vi "add rows_2 (SubVI).vi"(1 "array in":dbl[][](array[numeric])) -> (0 "array out":dbl[](array[numeric]))   [LabVIEW 2009]
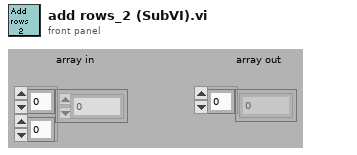
[diagram p1: front panel]
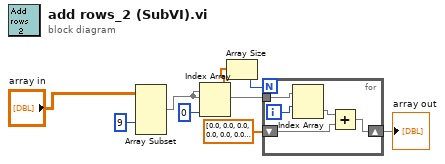
[diagram p0: block diagram]
diagram:
  n1 = Array Subset(array="array in", index (col)=9 ("index")) -> (w3:dbl[][])  [unwired: 3 in]
  n2 = Index Array(array=w3, index (col)=0 ("disabled index (col)")) -> (element=w5:dbl[])  [unwired: 1 in]
  n3 = Array Size(array=w5) -> (size(s)=w6:i32)
  n4 = for {
    N: w6 -> [_]
    tunnel: w3 -> [w13]
    shift-right: [w10] -> w1
    shift-left: dbl[] [0.0, 0.0, 0.0, 0.0, 0.0, 0.0, 0.0, 0.0, 0.0] -> [w9]
    i -> [w12]
    n5 = Index Array(array=w13, index (row)=w12) -> (element=w11:dbl[])  [unwired: 1 in]
    n6 = Add(x=w11, y=w9) -> (x+y=w10:dbl[])
  }
  "array out" <- w1
